vi "SR400 ReadCount.vi"(7 "Nb de période":i32=1 min=1 max=2000 step=1, 8 "error in (no error)":errorcluster, 9 "Compteur":u16(ring) items=["A", "B", "A+B"], 10 "AcqRef":refnum<vi>, 11 "VISA Port In":refnum<visa-resource-name>="GPIB0::23::INSTR") -> (0 "error out":errorcluster, 2 "Données":dbl[](array[numeric]), 3 "VISA Port Out":refnum<visa-resource-name>="GPIB0::23::INSTR", 5 "Status Code":u8)   [LabVIEW 2012]
uses:
  <vilib>/Utility/error.llb/DialogType.ctl
panel:
  out "Scan Lenght_ms":i32
  out "Dwell time":dbl=6.0 caption="\"Dwell Time\" (s)" min=0.002 max=6.0 step=0.001
  out "CounterPresT":dbl=0.001 caption="Counter T Preset (s)" min=1e-07 max=90000.0 step=1e-07 format="%#.7g"
  out "Acq en cours":bool caption="Acquisition\n en cours"
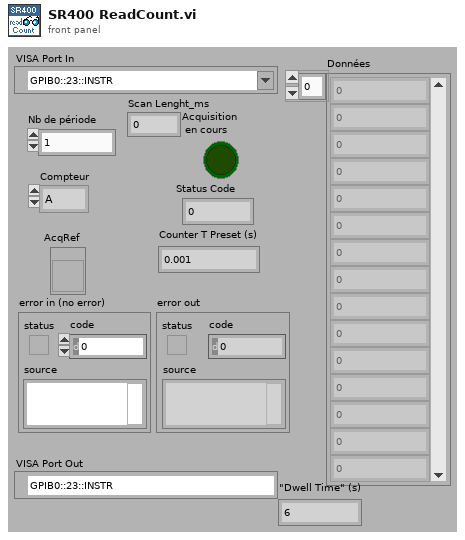
[diagram p1: front panel]
types:
  T1 = enum16{"Lit le Statut", "Init. les compteurs", "Attend fin du scan", "Lit les données", "Oper Incomplète"}
  T2 = typedef "DialogType.ctl" = u16
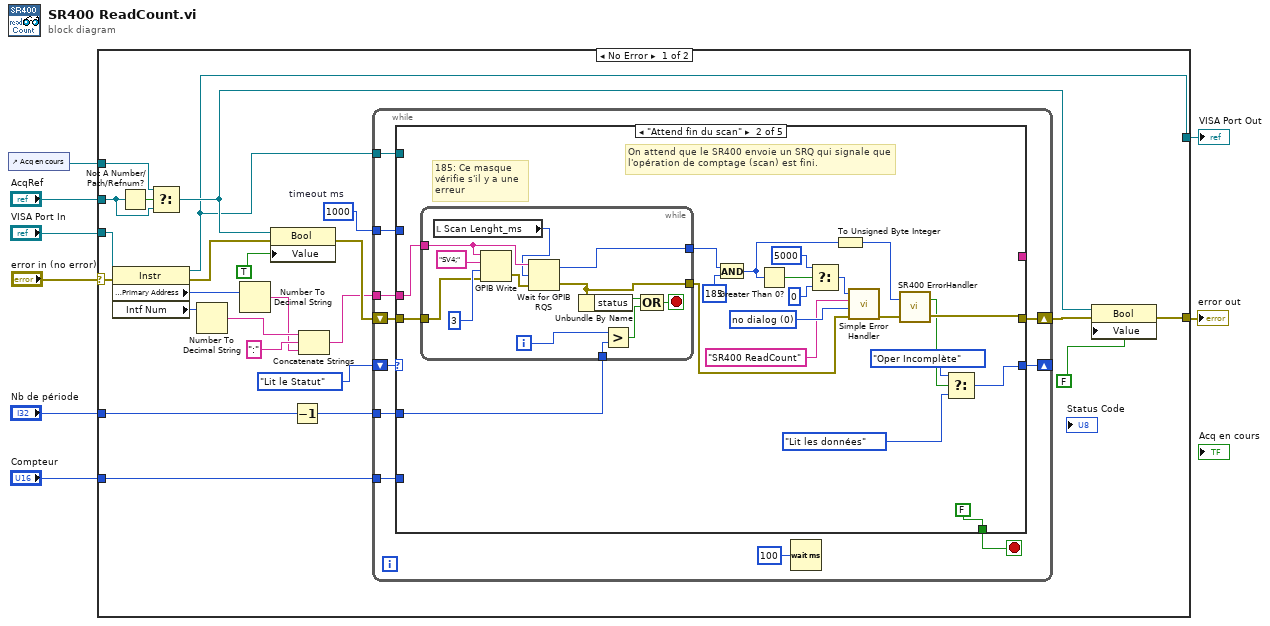
[diagram p0: block diagram]
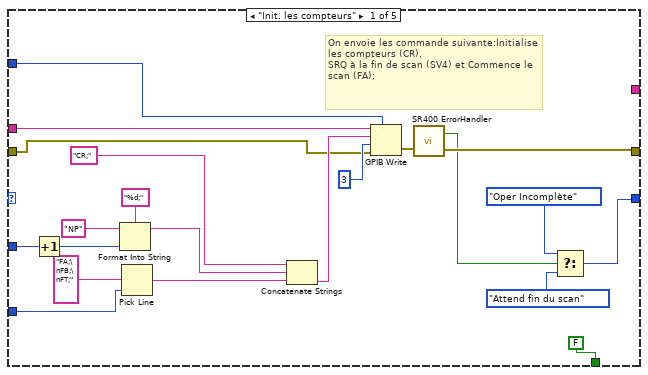
[diagram p2: hidden frame]
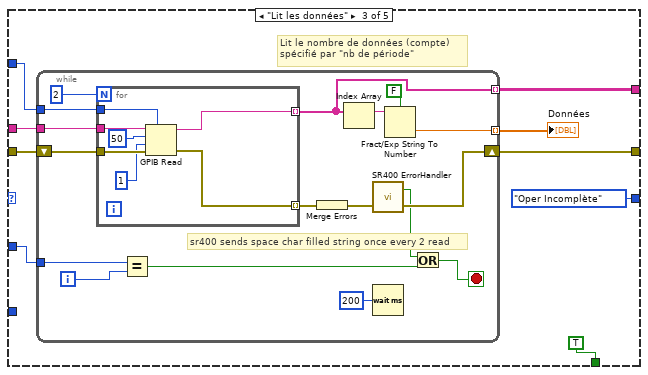
[diagram p3: hidden frame]
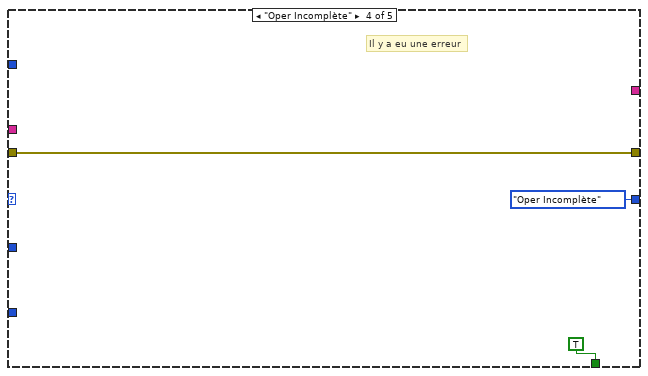
[diagram p4: hidden frame]
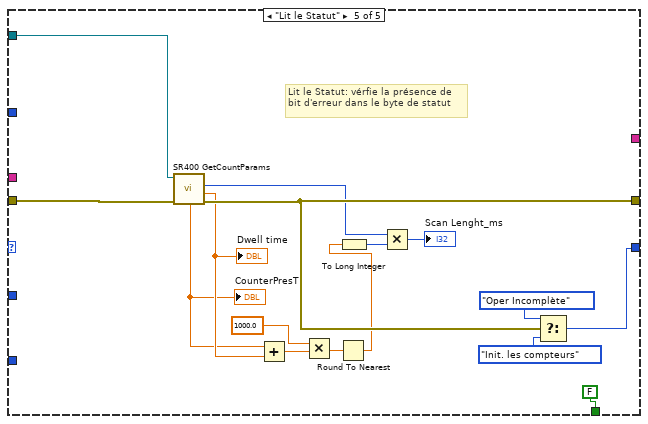
[diagram p5: hidden frame]
diagram:
  n1 = control-ref of="Acq en cours"() -> (w5:refnum<vi>)
  n2 = case shown="No Error" "error in (no error)" {
    selector: "error in (no error)" -> [w31 w152]
    tunnel: [w19 w152] -> w4
    tunnel: "VISA Port In" -> [w10 w151]
    tunnel: "Nb de période" -> [w21 _]
    tunnel: "AcqRef" -> [w27 _]
    tunnel: w5 -> [w26 _]
    tunnel: "Compteur" -> [w16 _]
    tunnel: [w9 w151] -> w1
    frame No Error {
      w30 = 1000  # timeout ms
      n3 = property class="Instr"(reference=w10, error in=w31) -> (reference out=w9:refnum<visa-resource-name>, error out=w25:errorcluster, "GPIB Settings:Primary Address"=w32:u16, "Intf Num"=w15:u16)
      n4 = Not A Number/Path/Refnum?(number/path/refnum=w27) -> (NaN/Path/Refnum?=w28:bool)
      n5 = Select(t=w26, s=w28, f=w27) -> (s? t:f=w17:refnum<vi>)
      n6 = Number To Decimal String(number=w15) -> (decimal integer string=w13:string)  [unwired: 1 in]
      n7 = Number To Decimal String(number=w32) -> (decimal integer string=w12:string)  [unwired: 1 in]
      n8 = property class="Bool"(reference=w17, error in=w25, "Value"=TRUE) -> (error out=w23:errorcluster)  [unwired: 1 out]
      n9 = Decrement(x=w21) -> (x-1=w20:i32)
      n10 = Concatenate Strings(w13, ":" ("string"), w12) -> (w11:string)
      n11 = while {
        tunnel: w11 -> [w43]
        tunnel: w30 -> [w41]
        shift-right: [w40] -> w18
        shift-left: w23 -> [w42]
        shift-right: [w36] -> _
        shift-left: T1."Lit le Statut" -> [w39]
        tunnel: w20 -> [w38]
        tunnel: w16 -> [w34]
        tunnel: w9 -> [w33]
        stop <- w37 stop-if-true
        n12 = case shown="\"Attend fin du scan\"" w39 {
          tunnel: w43 -> [w64 w68 w100 _ _]
          tunnel: w42 -> [w44 w67 w101 w132 w145]
          tunnel: w41 -> [w63 _ w105 _ _]
          tunnel: [w60 w84 w104 w132 w144] -> w40
          tunnel: [w58 w85 T1."Oper Incomplète" T1."Oper Incomplète" w148] -> w36
          tunnel: w38 -> [w52 w65 w107 _ _]
          tunnel: [FALSE ("Données lues") FALSE ("Données lues") TRUE ("Données lues") TRUE ("Données lues") FALSE ("Données lues")] -> w37
          tunnel: w34 -> [w53 _ _ _ _]
          tunnel: [_ _ w99 _ _] -> _
          tunnel: w33 -> [_ _ _ _ w146]
          frame "Init. les compteurs" {
            # "On envoie les commande suivante:Initialise les compteurs (CR),\nSRQ à la fin de scan (SV4) et Commence le scan (FA);"
            n13 = Increment(x=w52) -> (x+1=w49:i32)
            n14 = Format Into String(format string="%d;", initial string="NP", w49) -> (resulting string=w46:string)  [unwired: 1 in, 1 out]
            n15 = Pick Line(multi-line string="FA;\nFB;\nFT;" ("data"), line index=w53) -> (output string=w47:string)  [unwired: 1 in]
            n16 = Concatenate Strings("CR;" ("data"), w46, w47) -> (w50:string)
            n17 = GPIB Write(0:w64, 1:w50, 2:i16 3 ("mode (0)"), 3:w44, 4:w63) -> (6:w61:errorcluster)  [unwired: 1 out]
            n18 = call <userlib>:"SR400 ErrorHandler.vi"("error in (no error)"=w61) -> ("error out"=w60:errorcluster, "Erreur"=w59:bool)  [unwired: 1 in]
            n19 = Select(t=T1."Oper Incomplète", s=w59, f=T1."Attend fin du scan") -> (s? t:f=w58:T1)
          }
          frame "Attend fin du scan" {
            w75 = T2 0 items=["no dialog", "OK message", "continue or stop message", "OK message + warnings", "continue/stop + warnings"] ("type of dialog (OK msg:1)")
            # "185: Ce masque vérifie s'il y a une erreur"
            # "On attend que le SR400 envoie un SRQ qui signale que l'opération de comptage (scan) est fini."
            n20 = while {
              tunnel: [w93] -> w70
              tunnel: [w98] -> w69
              tunnel: w68 -> [w88]
              tunnel: w67 -> [w90]
              tunnel: w65 -> [w86]
              i -> [w94]
              stop <- w95 stop-if-true
              n21 = local read "Scan Lenght_ms"() -> (w87:i32)
              n22 = GPIB Write(0:w88, 1:"SV4;" ("data"), 2:i16 3 ("mode (0)"), 3:w90) -> (6:w89:errorcluster)  [unwired: 1 in, 1 out]
              n23 = Wait for GPIB RQS(2:w89, 3:w87, 4:w88) -> (0:w93:errorcluster, 1:w98:i16)
              n24 = Unbundle By Name(w93) -> ("status"=w97:bool)
              n25 = Greater?(x=w94, y=w86) -> (0:w96:bool)
              n26 = Compound Arithmetic op=OR(w97, w96) -> (w95:bool)
            }
            n27 = And(x=w69, y=i16 185) -> (x .and. y?=w73:i16)
            n28 = Greater Than 0?(x=w73) -> (x > 0?=w77:bool)
            n29 = Select(t=5000, s=w77, f=0) -> (s? t:f=w76:i32)
            n30 = To Unsigned Byte Integer(number=w73) -> (unsigned 8bit integer=w72:u8)
            n31 = call <vilib>:"Simple Error Handler.vi"("error code (no error:0)"=w76, "error source (\" \")"="SR400 ReadCount" ("[error source] (\" \")"), "type of dialog (OK msg:1)"=w75, "error in (no error)"=w70) -> ("error out"=w74:errorcluster)  [unwired: 1 in, 4 out]
            n32 = call <userlib>:"SR400 ErrorHandler.vi"("error in (no error)"=w74, "Status Code"=w72) -> ("error out"=w84:errorcluster, "Erreur"=w81:bool)
            n33 = Select(t=T1."Oper Incomplète", s=w81, f=T1."Lit les données") -> (s? t:f=w85:T1)
          }
          frame "Lit les données" {
            # "Lit le nombre de données (compte)\nspécifié par \"nb de période\""
            n34 = while {
              tunnel: w100 -> [w124]
              shift-right: [w115] -> w104
              shift-left: w101 -> [w123]
              tunnel: [w122] -> w106 mode=indexing
              tunnel: w107 -> [w120]
              tunnel: w105 -> [w118]
              tunnel: [w108] -> w99 mode=indexing
              i -> [w121]
              stop <- w119 stop-if-true
              # "sr400 sends space char filled string once every 2 read"
              n35 = for {
                N: 2 -> [_]
                tunnel: w124 -> [w131]
                tunnel: w123 -> [w130]
                tunnel: w118 -> [w127]
                tunnel: [w126] -> w116 mode=indexing
                tunnel: [w125] -> w108 mode=indexing
                n36 = GPIB Read(0:w131, 1:50 ("byte count"), 2:i16 1 ("mode (0)"), 3:w130, 4:w127) -> (5:w125:string, 7:w126:errorcluster)  [unwired: 1 out]
              }
              n37 = Equal?(x=w120, y=w121) -> (x = y?=w117:bool)
              n38 = Merge Errors(w116) -> (w109:errorcluster)
              n39 = Index Array(array=w108) -> (element=w110:string)  [unwired: 1 in]
              n40 = call <userlib>:"SR400 ErrorHandler.vi"("error in (no error)"=w109) -> ("error out"=w115:errorcluster, "Erreur"=w114:bool)  [unwired: 1 in]
              n41 = Wait (ms)(milliseconds to wait=u32 200) -> ()  [unwired: 1 out]
              n42 = Fract/Exp String To Number(use system decimal point (T)=FALSE, string=w110) -> (number=w122:dbl)  [unwired: 2 in, 1 out]
              n43 = Or(x=w114, y=w117) -> (x .or. y?=w119:bool)
            }
            "Données" <- w106
          }
          frame "Oper Incomplète" {
            # "Il y a eu une erreur"
          }
          frame "Lit le Statut" {
            # "Lit le Statut: vérfie la présence de bit d'erreur dans le byte de statut"
            n44 = call <userlib>:"SR400 GetCountParams.vi"("error in (no error)"=w145, "VISA Port In"=w146) -> ("error out"=w144:errorcluster, "Dwell time"=w143:dbl, "Nb de période"=w139:i32, "CounterPresT"=w142:dbl)  [unwired: 3 in, 3 out]
            "CounterPresT" <- w142
            "Dwell time" <- w143
            n45 = Add(x=w142, y=w143) -> (x+y=w141:dbl)
            n46 = Multiply(x=1000.0, y=w141) -> (x*y=w138:dbl)
            n47 = Round To Nearest(number=w138) -> (nearest integer value=w137:dbl)
            n48 = To Long Integer(number=w137) -> (32bit integer=w136:i32)
            n49 = Multiply(x=w139, y=w136) -> (x*y=→"Scan Lenght_ms":i32)
            n50 = Select(t=T1."Oper Incomplète", s=w144, f=T1."Init. les compteurs") -> (s? t:f=w148:T1)
          }
        }
        n51 = Wait (ms)(milliseconds to wait=u32 100) -> ()  [unwired: 1 out]
      }
      n52 = property class="Bool"(reference=w17, error in=w18, "Value"=FALSE) -> (error out=w19:errorcluster)  [unwired: 1 out]
    }
    frame Error {
    }
  }
  "error out" <- w4
  "VISA Port Out" <- w1
